vi "Create Default Attributes.vi"(5 "Unique ID":string, 7 "Process Executive Ref":refnum<data-value>, 11 "Stop Low Pressure Wax in":refnum<class "Stop Low Pressure Wax.lvclass">) -> (3 "Stop Low Pressure Wax out":refnum<class "Stop Low Pressure Wax.lvclass">)   [LabVIEW 2019, in "Stop Low Pressure Wax.lvclass"]
uses:
  <vilib>/gpm_packages/@cs/Car-wash/Source/Process Steps/Stop Low Pressure Wax/Stop Low Pressure Wax.lvclass
  <vilib>/gpm_packages/@cs/test-executive/Source/Test Executive/ITestExecutive/ITest Executive.lvclass
  7a3d9f99-7b50-4469-b609-027c910f6b26.vi
  <vilib>/Utility/error.llb/Error Cluster From Error Code.vi
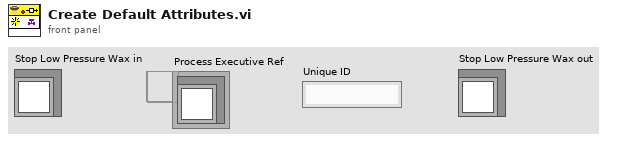
[diagram p1: front panel]
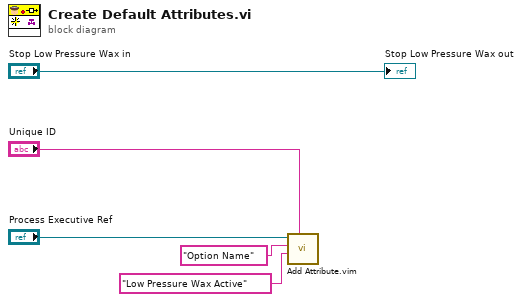
[diagram p0: block diagram]
diagram:
  n1 = call "Add Attribute.vim"("ID"="Unique ID", "Attribute"="Low Pressure Wax Active" ("Item Name"), "Attribute Name"="Option Name" ("Item Name"), "Test Executive Ref"="Process Executive Ref") -> ()  [unwired: 4 in, 4 out]
  "Stop Low Pressure Wax out" <- "Stop Low Pressure Wax in"
